vi "Init Actor Core.vi"(8 "error in (no error)":errorcluster, 11 "Measure Object in":refnum<class "Combined Measurement.lvclass">) -> (0 "error out":errorcluster, 3 "Measure Object out":refnum<class "Combined Measurement.lvclass">)   [LabVIEW 2021, in "Combined Measurement.lvclass"]
uses:
  Combined Measurement.lvclass
  C:/GitHub/LabActor/Template Module/Template Module.lvclass
  NHMFL_Core/Libraries/Instruments/Results/Acquired Result/Acquired Result.lvclass
  Template Module/Template Module.lvclass/Template Module.ctl
  Combined Measurement.lvclass/Combined Measurement.ctl
  Template Module/Read Name.vi
  Continuous Recorder Actor/Continuous Recorder Actor.lvclass
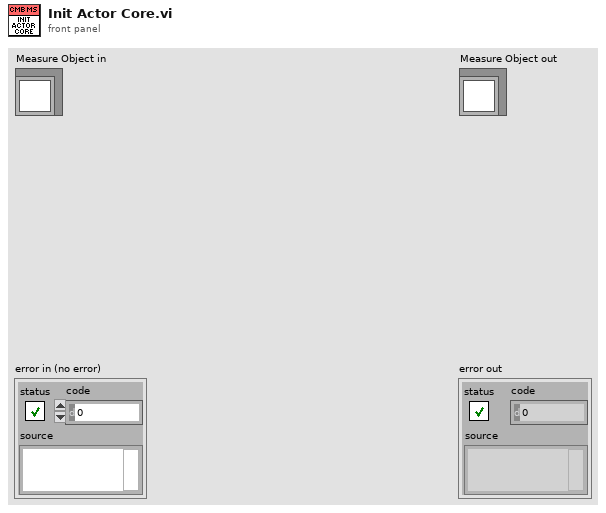
[diagram p1: front panel]
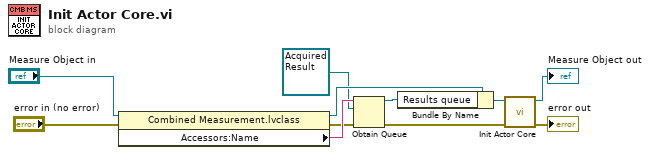
[diagram p0: block diagram]
diagram:
  n1 = property class="Combined Measurement.lvclass"(reference="Measure Object in", error in="error in (no error)") -> (reference out=w7:refnum<class "Combined Measurement.lvclass">, error out=w4:errorcluster, "Accessors:Name"=w6:string)
  n2 = Obtain Queue(name (unnamed)=w6, element data type=refnum<class "Acquired Result.lvclass"> refnum ("Acquired Result.lvclass"), error in (no error)=w4) -> (queue out=w1:refnum<queue>, error out=w3:errorcluster)  [unwired: 2 in, 1 out]
  n3 = Bundle By Name(cluster=w7, "Results queue"=w1) -> (w2:refnum<class "Combined Measurement.lvclass">)
  n4 = call-parent "Init Actor Core.vi"("error in (no error)"=w3, "Measure Object in"=w2) -> ("error out"=→"error out":errorcluster, "Measure Object out"=→"Measure Object out":refnum<class "Combined Measurement.lvclass">)  [unwired: 8 in]
